vi "Start Wfms.vi"(8 "error in (no error)":errorcluster, 11 "Channel Manager in":refnum<class "Channel Manager.lvclass">) -> (0 "error out":errorcluster, 3 "Channel Manager out":refnum<class "Channel Manager.lvclass">)   [LabVIEW 2024, in "Embedded TDMS Logger Engine.lvlib" / "Channel Manager.lvclass"]
doc: "Gets our waveforms references and opens a session with the waveforms and then stores the reference in their corresponding channels."
uses:
  Channel Manager.lvclass
  Channel Manager.lvclass/Channel Manager.ctl
  Shared/File Classes/File/File.lvclass
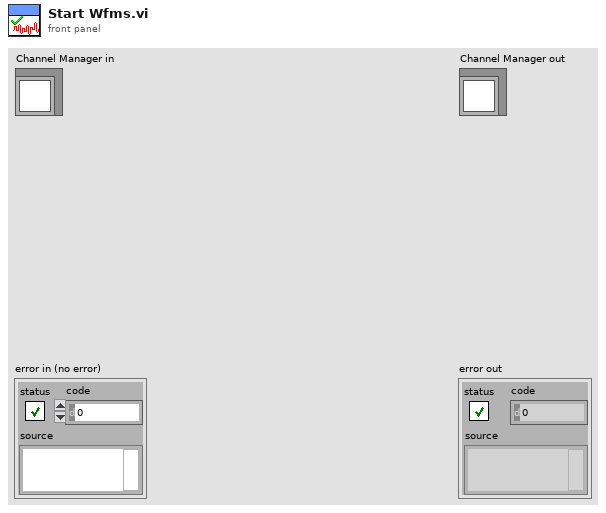
[diagram p1: front panel]
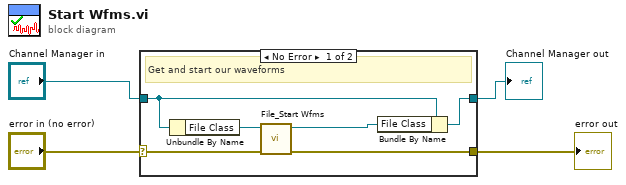
[diagram p0: block diagram]
diagram:
  n1 = case shown="No Error" "error in (no error)" {
    selector: "error in (no error)" -> [w5 w12]
    tunnel: [w8 w12] -> w3
    tunnel: [w10 w11] -> w1
    tunnel: "Channel Manager in" -> [w7 w11]
    frame No Error {
      # "Get and start our waveforms"
      n2 = Unbundle By Name(w7) -> ("File Class"=w6:refnum<class "File.lvclass">)
      n3 = call-dynamic "File_Start Wfms.vi"("error in (no error)"=w5, "File in"=w6) -> ("error out"=w8:errorcluster, "File out"=w9:refnum<class "File.lvclass">)  [unwired: 8 in]
      n4 = Bundle By Name(cluster=w7, "File Class"=w9) -> (w10:refnum<class "Channel Manager.lvclass">)
    }
    frame Error {
    }
  }
  "error out" <- w3
  "Channel Manager out" <- w1
